vi "General-ConvertArray2OneDimension.vi"(1 "Input Array":dbl[][](array[numeric])) -> (0 "Output Array":dbl[](array[numeric]))   [LabVIEW 2010]
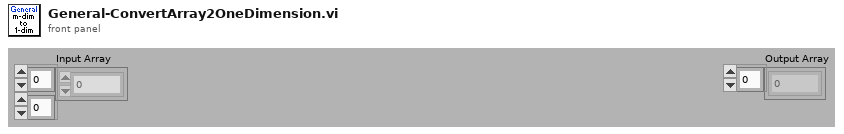
[diagram p1: front panel]
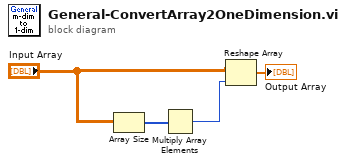
[diagram p0: block diagram]
diagram:
  n1 = Array Size(array="Input Array") -> (size(s)=w3:i32[])
  n2 = Multiply Array Elements(1:w3) -> (0:w4:i32)
  n3 = Reshape Array("Input Array", w4) -> (→"Output Array":dbl[])
